vi "Write planetName.vi"(8 "error in (no error)":errorcluster, 10 "planetName":T1, 11 "Planet in":refnum<class "Planet.lvclass">) -> (0 "error out":errorcluster, 3 "Planet out":refnum<class "Planet.lvclass">)   [LabVIEW 2014, in "TCSDataDefinitions.lvlib" / "TCSCommand.lvlib" / "TargetConfiguration.lvlib" / "Target.lvlib" / "Planet.lvclass"]
uses:
  Planet.lvclass
  Enumerations/PlanetNameValues.ctl
  Planet.lvclass/Planet.ctl
  Target.lvlib
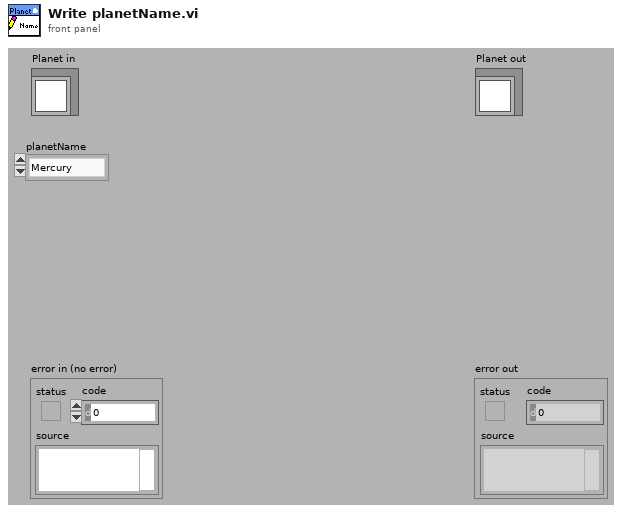
[diagram p1: front panel]
types:
  T1 = typedef "TCSDataDefinitions.lvlib/TCSCommand.lvlib/TargetConfiguration.lvlib/Target.lvlib/PlanetNameValues.ctl" = enum16{"Mercury", "Venus", "Moon", "Mars", "Jupiter", "Saturn", "Uranus", "Neptune", "Pluto"}
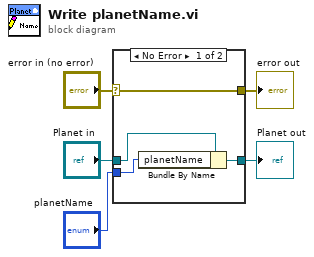
[diagram p0: block diagram]
diagram:
  n1 = case shown="No Error" "error in (no error)" {
    selector: "error in (no error)" -> [w9 w10]
    tunnel: [w9 w10] -> w4
    tunnel: [w7 w11] -> w2
    tunnel: "Planet in" -> [w8 w11]
    tunnel: "planetName" -> [w6 _]
    frame No Error {
      n2 = Bundle By Name(cluster=w8, "planetName"=w6) -> (w7:refnum<class "Planet.lvclass">)
    }
    frame Error {
    }
  }
  "error out" <- w4
  "Planet out" <- w2
